vi "_GetStatusByte.vi"(8 "error in":errorcluster, 11 "Instrument Channel":string="GPIB/0:4,0") -> (0 "error out":errorcluster, 1 "MAV bit":bool, 2 "Status Byte":i16, 3 "Instrument Channel out":string="GPIB/0:4,0")   [LabVIEW 2020, in "FCR100.lvlib"]
doc: "Retrieves the status byte and parses out the Message Available Bit (MAV). \n\nThis is very fast for GPIB, and normal query speed for other busses."
uses:
  FCR100.lvlib
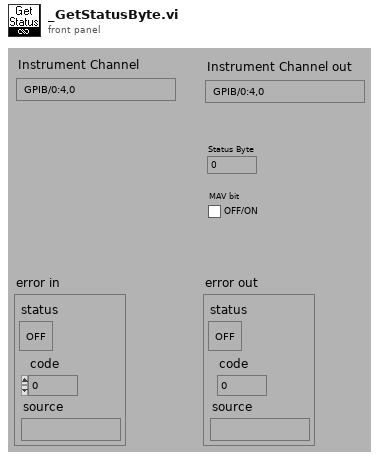
[diagram p1: front panel]
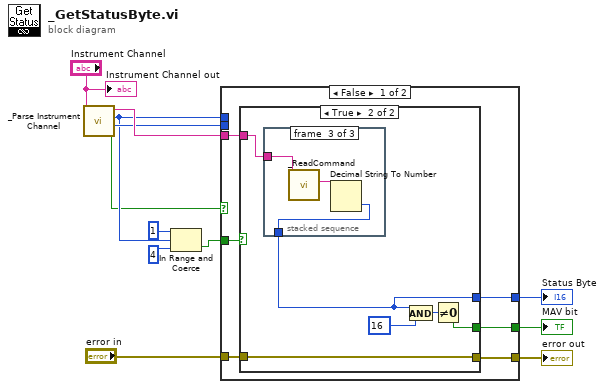
[diagram p0: block diagram]
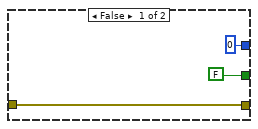
[diagram p2: hidden frame]
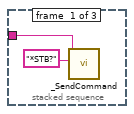
[diagram p3: hidden frame]
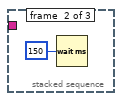
[diagram p4: hidden frame]
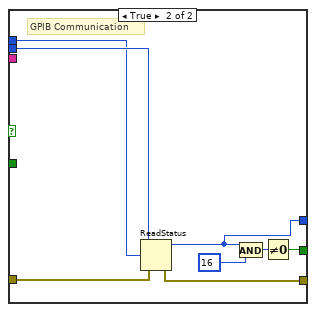
[diagram p5: hidden frame]
diagram:
  n1 = call "_Parse Instrument Channel.vi"("Instrument Channel"="Instrument Channel") -> ("T - GPIB, F - RS232"=w1:bool, "Hardware Address"=w3:i32, "Instrument Address"=w2:i16, "Instrument Channel out"=w7:string)  [unwired: 6 in, 1 out]
  n2 = In Range and Coerce(upper limit=1, x=w2, lower limit=4) -> (In Range?=w4:bool)  [unwired: 1 out]
  n3 = case shown="False" w1 {
    tunnel: w4 -> [w16 _]
    tunnel: "error in" -> [w18 w41]
    tunnel: [w17 w40] -> w11
    tunnel: [w15 w38] -> w10
    tunnel: [w14 w36] -> w9
    tunnel: w7 -> [w13 _]
    tunnel: w3 -> [_ w35]
    tunnel: w2 -> [_ w34]
    frame False {
      n4 = case shown="True" w16 {
        tunnel: w18 -> [w21 w27]
        tunnel: [w21 w27] -> w17
        tunnel: [FALSE w22] -> w15
        tunnel: [0 w23] -> w14
        tunnel: w13 -> [_ w26]
        frame False {
        }
        frame True {
          n5 = stacked-sequence {
            tunnel: w26 -> [w29 _ w33]
            tunnel: [_ _ w31] -> w23
            frame #0 {
              n6 = call "_SendCommand.vi"("Command"="*STB?", "Instrument Channel"=w29) -> ()  [unwired: 8 in, 2 out]
            }
            frame #1 {
              n7 = Wait (ms)(milliseconds to wait=150) -> ()  [unwired: 1 out]
            }
            frame #2 {
              n8 = call "_ReadCommand.vi"("Instrument Channel"=w33) -> ("Response"=w32:string)  [unwired: 8 in, 2 out]
              n9 = Decimal String To Number(string=w32) -> (number=w31:i32)  [unwired: 2 in, 1 out]
            }
          }
          n10 = And(x=w23, y=u16 16) -> (x .and. y?=w24:i32)
          n11 = Not Equal To 0?(x=w24) -> (x != 0?=w22:bool)
        }
      }
    }
    frame True {
      # "GPIB Communication"
      n12 = ReadStatus(3:w41, 4:w34, 5:w35) -> (0:w40:errorcluster, 2:w36:i16)  [unwired: 1 out]
      n13 = And(x=w36, y=u16 16) -> (x .and. y?=w37:u16)
      n14 = Not Equal To 0?(x=w37) -> (x != 0?=w38:bool)
    }
  }
  "error out" <- w11
  "MAV bit" <- w10
  "Status Byte" <- w9
  "Instrument Channel out" <- "Instrument Channel"
